vi "Load Accounts Data.vi"(8 "error in":errorcluster) -> (0 "error out":errorcluster, 3 "Accounts":T1[](array[typedef]))   [LabVIEW 2019, in "Configuration Database.lvlib"]
doc: "Reads txt file to load accounts data."
uses:
  Configuration Database.lvlib
  Typedefs/Account.ctl
panel:
  # "[Covers: CD1A]"
  # "[Covers: CD1B]"
  # "[Covers: CD1C]"
  # "[Covers: CD1D]"
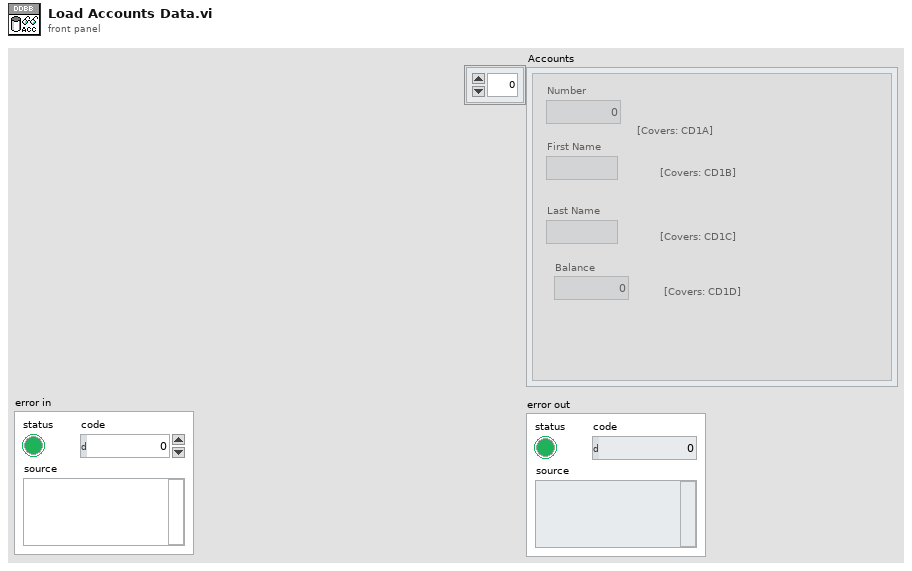
[diagram p1: front panel]
types:
  T1 = typedef "Configuration Database.lvlib/Account.ctl" = cluster{"Number":i32, "First Name":string, "Last Name":string, "Balance":dbl}
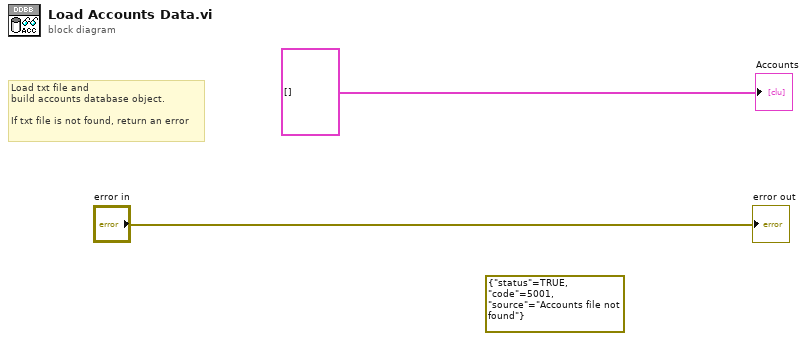
[diagram p0: block diagram]
diagram:
  (unwired) errorcluster {"status"=TRUE, "code"=5001, "source"="Accounts file not found"} ("error in")
  # "Load txt file and \nbuild accounts database object. \n\nIf txt file is not found, return an error"
  "Accounts" <- T1[] [] ("Array")
  "error out" <- "error in"
